vi "ESP301_Read_Position_loop.vi"(10 "axisNumber":i32=1, 11 "COM_PORT":string="COM12") -> (0 "errstring":string, 1 "MD":bool, 2 "Motor_status":bool, 3 "Position":dbl)   [LabVIEW 2019]
uses:
  Newport.ESP301.CommandInterface
panel:
  in  "stop":bool
  out "MD":i32
  out "errstring 3":string
  out "errstring 2":string
  out "MO_Get":i32
  out "TP":i32
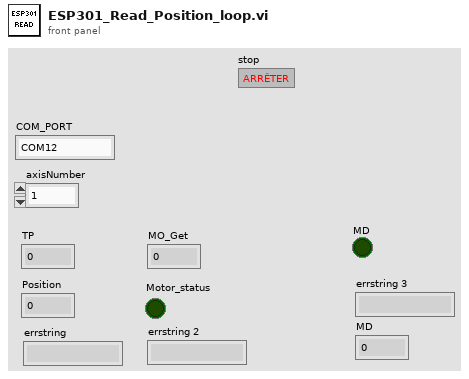
[diagram p1: front panel]
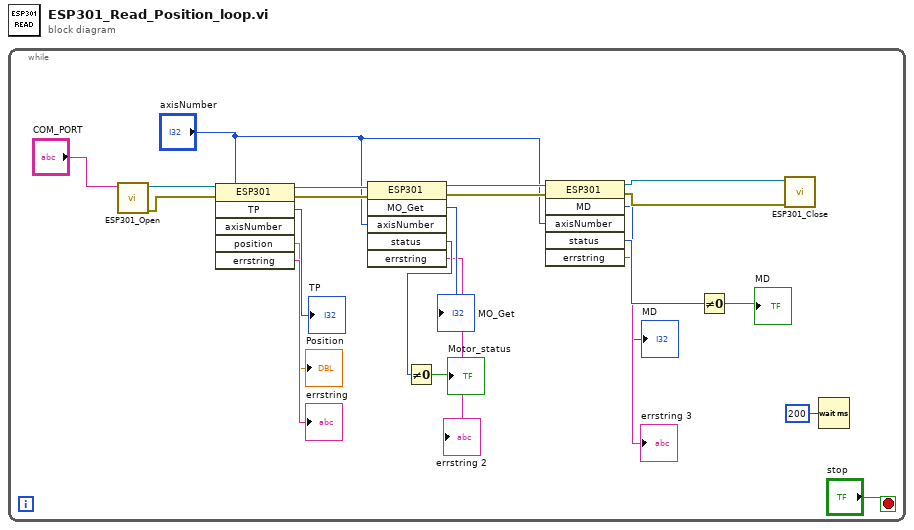
[diagram p0: block diagram]
diagram:
  n1 = while {
    stop <- "stop" stop-if-true
    n2 = call "ESP301_Open.vi"("strDeviceKey"="COM_PORT") -> ("sortie d'erreur"=w20:errorcluster, "référence en sortie"=w21:refnum<k24>)  [unwired: 9 in]
    n3 = invoke on="Nœud de méthode" class="ESP301" method="TP"(reference=w21, error in=w20, "axisNumber"="axisNumber") -> (reference out=w23:refnum<k24>, error out=w22:errorcluster, "TP"=→"TP":i32, "position"=→"Position":dbl, "errstring"=→"errstring":string)  [unwired: 3 in, 1 out]
    n4 = invoke on="Nœud de méthode" class="ESP301" method="MO_Get"(reference=w23, error in=w22, "axisNumber"="axisNumber") -> (reference out=w11:refnum<k24>, error out=w10:errorcluster, "MO_Get"=→"MO_Get":i32, "status"=w15:i32, "errstring"=→"errstring 2":string)  [unwired: 3 in, 1 out]
    n5 = Not Equal To 0?(x=w15) -> (x != 0?=→"Motor_status":bool)
    n6 = invoke on="Nœud de méthode" class="ESP301" method="MD"(reference=w11, error in=w10, "axisNumber"="axisNumber") -> (reference out=w9:refnum<k24>, error out=w8:errorcluster, "MD"=→"MD":i32, "status"=w6:i32, "errstring"=→"errstring 3":string)  [unwired: 3 in, 1 out]
    n7 = Not Equal To 0?(x=w6) -> (x != 0?=→"MD":bool)
    n8 = call "ESP301_Close.vi"("entrée d'erreur (pas d'erreur)"=w8, "référence"=w9) -> ()  [unwired: 9 in, 1 out]
    n9 = Wait (ms)(milliseconds to wait=u32 200 ("attente (ms)")) -> ()  [unwired: 1 out]
  }
